vi "SubPanel_RFBlock_Panel_Rev11_v2.vi"(2 "error input":errorcluster, 3 "RF Block Input Array":T1[](array[typedef])) -> (0 "error output":errorcluster, 1 "RF Block Output Array":T1[](array[typedef]))   [LabVIEW 2019]
uses:
  Controls/RFBlockControl.ctl
panel:
  out "RF Block Output Echo":T1[](array[typedef])
  in  "VISA resource name":refnum<visa-resource-name>
  in  "Apply Configuration":bool
  in  "Frequency (GHz)":dbl
  in  "Power (dBm)":dbl
  out "Frequency (GHz) Output":dbl
  out "Power (dBm) Output":dbl
  in  "Power On?":bool
  in  "EXIT SUBVI":bool
  # "Instructions\nSelect Resource Under Name\nPower it on\nProvide the Frequency and Power desired\nPress \"Apply\"\nSee the output on the Echo above. If there are multiple devices configured, there will be multiple elements in the array"
  # "Nothing to see behind here"
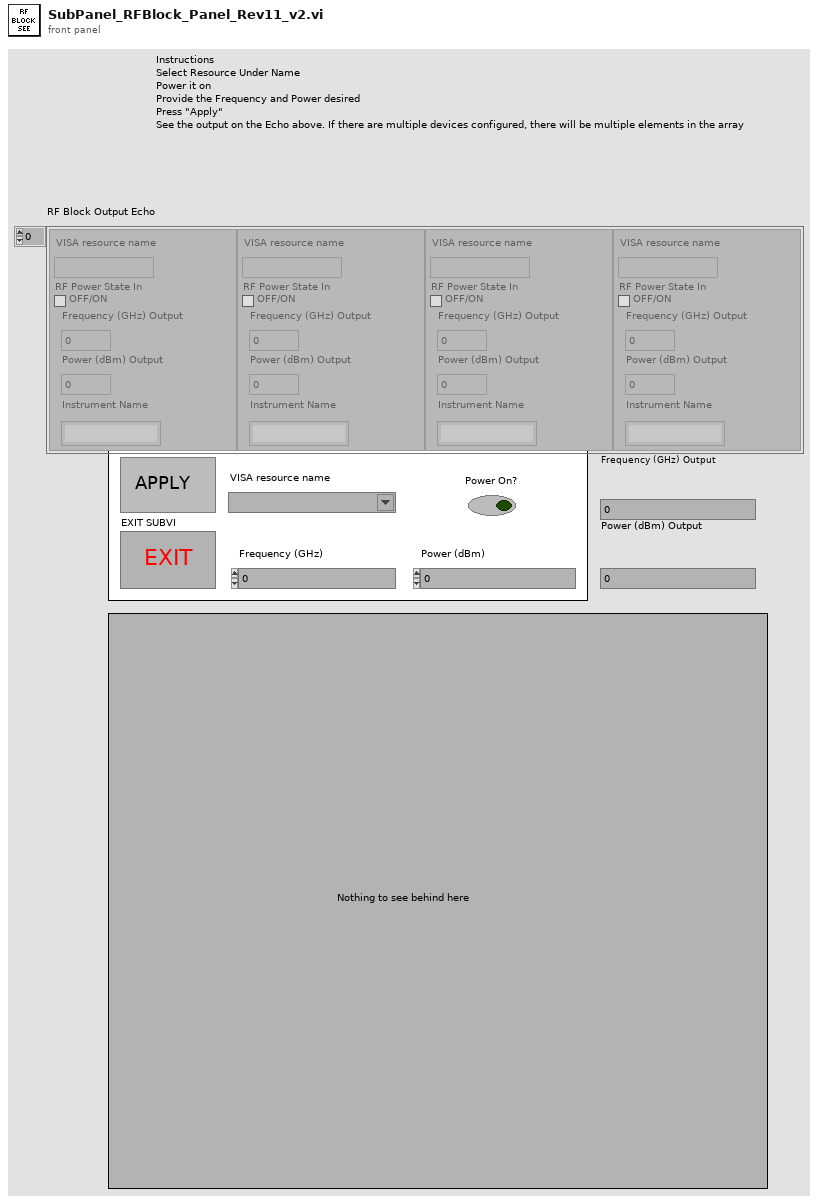
[diagram p1: front panel]
types:
  T1 = typedef "RFBlockControl.ctl" = cluster{"VISA resource name":refnum<visa-resource-name>, "RF Power State In":bool, "Frequency (GHz) Output":dbl, "Power (dBm) Output":dbl, "Instrument Name":string}
  T2 = cluster{"VISA resource name":refnum<visa-resource-name>, "Boolean out":bool, "Frequency (GHz) Output":dbl, "Power (dBm) Output":dbl}
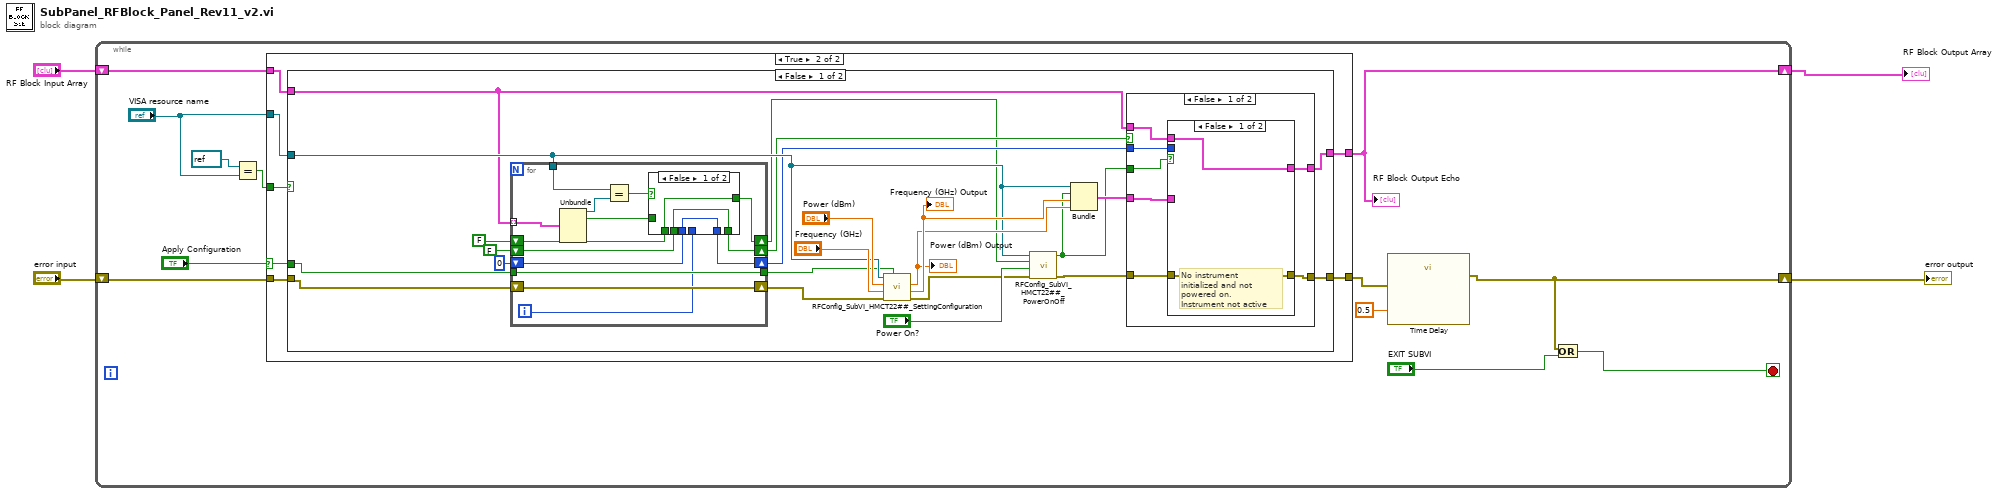
[diagram p0: block diagram]
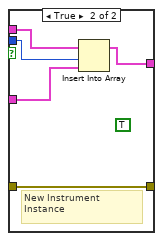
[diagram p3: hidden frame]
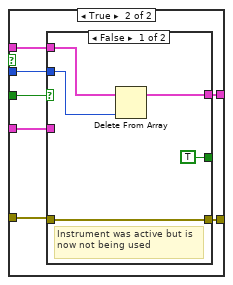
[diagram p4: hidden frame]
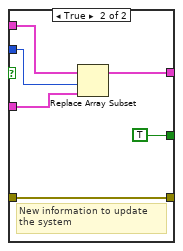
[diagram p5: hidden frame]
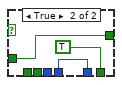
[diagram p6: hidden frame]
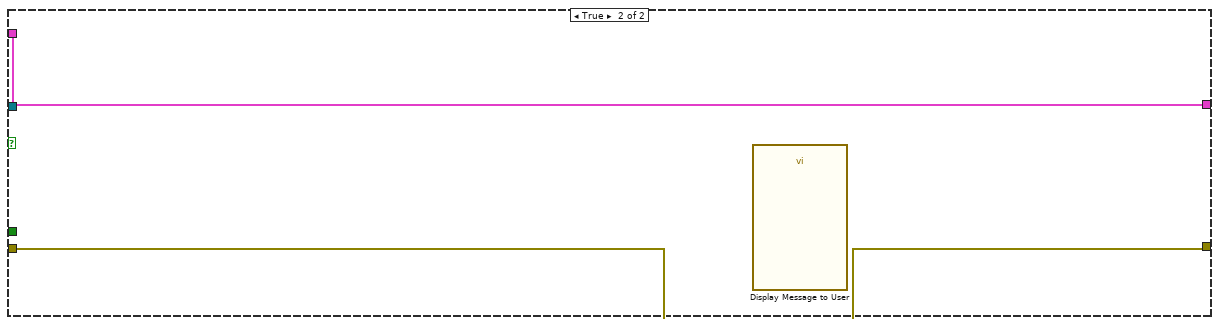
[diagram p7: hidden frame]
diagram:
  n1 = while {
    shift-right: [w7] -> w3
    shift-left: "error input" -> [w14]
    shift-right: [w8] -> w1
    shift-left: "RF Block Input Array" -> [w9]
    stop <- w5 stop-if-true
    n2 = Equal?(x=refnum<visa-resource-name> refnum ("VISA resource name"), y="VISA resource name") -> (x = y?=w10:bool)
    n3 = case shown="True" "Apply Configuration" {
      selector: "Apply Configuration" -> [_ w22]
      tunnel: "VISA resource name" -> [_ w25]
      tunnel: [w18 w24] -> w13
      tunnel: w14 -> [w18 w23]
      tunnel: w10 -> [_ w21]
      tunnel: w9 -> [w17 w20]
      tunnel: [w17 w19] -> w8
      frame False {
      }
      frame True {
        n4 = case shown="False" w21 {
          tunnel: w25 -> [w40 _]
          tunnel: [w32 w102] -> w24
          tunnel: w23 -> [w42 w102]
          tunnel: w22 -> [w29 _]
          tunnel: w20 -> [w37 w101]
          tunnel: [w30 w101] -> w19
          frame False {
            n5 = for {
              tunnel: w37 -> [w94] mode=indexing
              shift-right: [w88] -> w41
              shift-left: w42 -> [w88]
              tunnel: w40 -> [w92]
              shift-right: [w89] -> w35
              shift-left: FALSE -> [w90]
              shift-right: [w83] -> w34
              shift-left: 0 -> [w84]
              tunnel: w29 -> [w87]
              tunnel: [w87] -> w28
              shift-right: [w81] -> w26
              shift-left: FALSE -> [w85]
              i -> [w82]
              n6 = Unbundle(w94) -> ("VISA resource name"=w93:refnum<visa-resource-name>, "RF Power State In"=w86:bool)  [unwired: 3 out]
              n7 = Equal?(x=w92, y=w93) -> (x = y?=w91:bool)
              n8 = case shown="False" w91 {
                tunnel: w90 -> [w97 _]
                tunnel: [w97 TRUE] -> w89
                tunnel: w86 -> [_ w98]
                tunnel: w85 -> [w95 _]
                tunnel: w84 -> [w96 _]
                tunnel: [w96 w99] -> w83
                tunnel: w82 -> [_ w99]
                tunnel: [w95 w98] -> w81
                frame False {
                }
                frame True {
                }
              }
            }
            n9 = call "RFConfig_SubVI_HMCT22##_SettingConfiguration.vi"("Apply Configurations"=w28, "error in (no error)"=w41, "Frequency (GHz)"="Frequency (GHz)", "Power (dBm)"="Power (dBm)", "VISA Refnum in"=w40) -> ("error out"=w45:errorcluster, "Frequency (GHz) Output"=w44:dbl, "Power (dBm) Output"=w43:dbl)  [unwired: 4 in]
            "Frequency (GHz) Output" <- w44
            "Power (dBm) Output" <- w43
            n10 = call "RFConfig_SubVI_HMCT22##_PowerOnOff.vi"("error in (no error)"=w45, "Power On?"="Power On?", "Boolean in"=w26, "VISA Refnum in"=w40) -> ("error out"=w33:errorcluster, "Boolean out"=w31:bool)  [unwired: 6 in]
            n11 = Bundle("VISA resource name"=w40, "Boolean out"=w31, "Frequency (GHz) Output"=w44, "Power (dBm) Output"=w43) -> (w36:T2)  [unwired: 1 in]
            n12 = case shown="False" w35 {
              tunnel: w37 -> [w54 w65]
              tunnel: w36 -> [w53 w63]
              tunnel: w34 -> [w52 w66]
              tunnel: w33 -> [w49 w68]
              tunnel: [w50 w69] -> w32
              tunnel: w31 -> [w55 w67]
              tunnel: [w51 w64] -> w30
              frame False {
                n13 = case shown="False" w55 {
                  tunnel: w54 -> [w56 w62]
                  tunnel: w53 -> [_ w61]
                  tunnel: w52 -> [_ w60]
                  tunnel: [w56 w59] -> w51
                  tunnel: [w57 w58] -> w50
                  tunnel: w49 -> [w57 w58]
                  frame False {
                    # "No instrument initialized and not powered on. Instrument not active"
                  }
                  frame True {
                    (unwired) TRUE
                    # "New Instrument Instance"
                    n14 = Insert Into Array(array=w62, index=w60, new element=w61) -> (w59:T1[])
                  }
                }
              }
              frame True {
                n15 = case shown="False" w67 {
                  tunnel: [w74 w80] -> w69
                  tunnel: w68 -> [w74 w80]
                  tunnel: w66 -> [w73 w78]
                  tunnel: w65 -> [w72 w79]
                  tunnel: [w71 w76] -> w64
                  tunnel: w63 -> [_ w77]
                  tunnel: [TRUE TRUE] -> _
                  frame False {
                    # "Instrument was active but is now not being used"
                    n16 = Delete From Array(array=w72, index=w73) -> (array with subset deleted=w71:T1[])  [unwired: 1 in, 1 out]
                  }
                  frame True {
                    # "New information to update the system"
                    n17 = Replace Array Subset(array=w79, new element=w77, index=w78) -> (w76:T1[])
                  }
                }
              }
            }
          }
          frame True {
            n18 = call "Display Message to User"() -> ()  [unwired: 10 in, 2 out]
          }
        }
      }
    }
    "RF Block Output Echo" <- w8
    n19 = call "Time Delay"("error in (no error)"=w13, "Delay Time (s)"=0.5) -> ("error out"=w7:errorcluster)  [unwired: 9 in]
    n20 = Or(x=w7, y="EXIT SUBVI") -> (x .or. y?=w5:bool)
  }
  "error output" <- w3
  "RF Block Output Array" <- w1
